vi "Teleop.vi"(10 "Match Info":T1={"Autonomous Elapsed Seconds"=0.0, "TeleOp Elapsed Seconds"=0.0, "Disabled Elapsed Seconds"=0.0, "Visited Autonomous"=FALSE, "Visited TeleOp"=FALSE, "Visited Disabled"=FALSE, "Autonomous Settings"={"Autonomous Style"=enum."Independent", "VI Refnum"=refnum}}, 11 "Call Context":T2) -> ()   [LabVIEW 2017]
doc: "This VI is called for each TeleOp packet received from the DS where the robot is not disabled. It is often used to read from the joysticks and update I/O or to update setpoints for timed control loops. It should complete and return within 20 milliseconds or it may miss DS packets."
uses:
  <vilib>/Rock Robotics/WPI/DriverStation/WPI_DriverStationDerivedRobotMode.ctl
  <vilib>/Rock Robotics/WPI/DriverStation/WPI_DriverStationMatch Info.ctl
  <vilib>/Rock Robotics/WPI/Utilities/WPI_GetSetVariantRefNum.vi
  Globals/Driver Controller Inputs.vi
  Globals/Manipulator Controller Inputs.vi
  Globals/Robot Global Data.vi
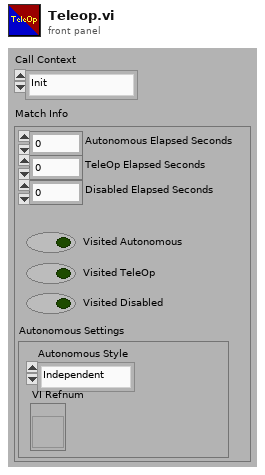
[diagram p1: front panel]
types:
  T1 = typedef "WPI_DriverStationMatch Info.ctl" = cluster{"Autonomous Elapsed Seconds":dbl, "TeleOp Elapsed Seconds":dbl, "Disabled Elapsed Seconds":dbl, "Visited Autonomous":bool, "Visited TeleOp":bool, "Visited Disabled":bool, "Autonomous Settings":cluster{"Autonomous Style":enum16{"Iterative", "Independent"}, "VI Refnum":refnum<vi>}}
  T2 = typedef "WPI_DriverStationDerivedRobotMode.ctl" = enum16{"Init", "Execute", "Stop"}
  T3 = typedef "WPI_JoystickDevRef.ctl" = cluster{"Device":T4}
  T4 = typedef "WPI_JoystickDeviceEnum.ctl" = enum16{"USB 0", "USB 1", "USB 2", "USB 3", "USB 4", "USB 5"}
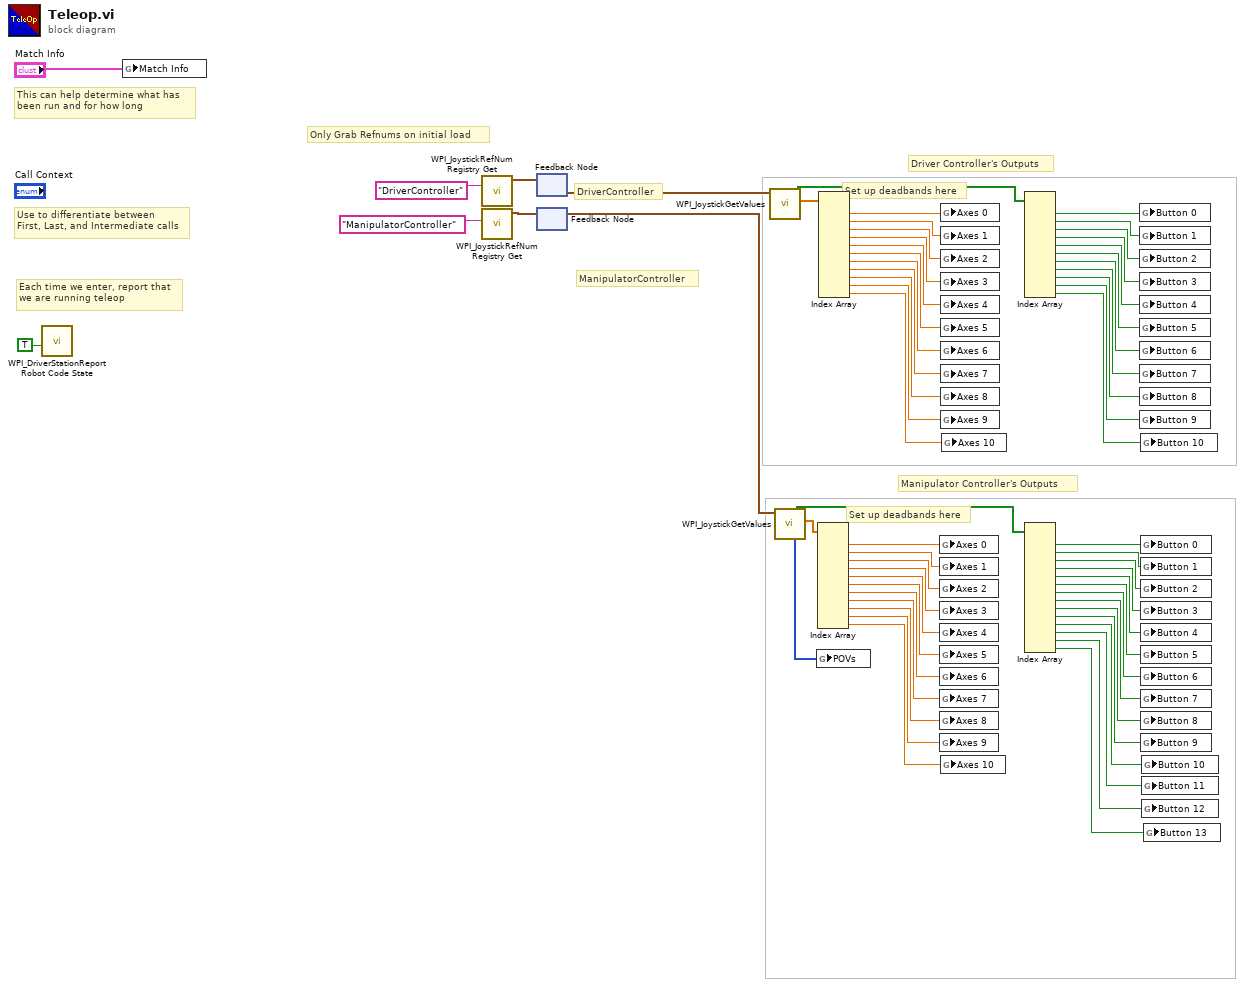
[diagram p0: block diagram]
diagram:
  # "ManipulatorController"
  # "DriverController"
  # "Only Grab Refnums on initial load"
  # "Set up deadbands here"
  # "Set up deadbands here"
  # "Driver Controller's Outputs"
  # "Manipulator Controller's Outputs"
  # "Each time we enter, report that\nwe are running teleop"
  # "Use to differentiate between\nFirst, Last, and Intermediate calls"
  # "This can help determine what has\nbeen run and for how long"
  n1 = call <vilib>:"WPI_DriverStationReport Robot Code State.vi"("TeleOp"=TRUE ("Autonomous")) -> ()  [unwired: 10 in, 1 out]
  n2 = global write "Robot Global Data.vi" "Match Info"("Match Info") -> ()
  n3 = call <vilib>:"WPI_JoystickRefNum Registry Get.vi"("refnum name"="DriverController") -> ("JoystickDevRef"=w9:T3)  [unwired: 1 in, 9 out]
  n4 = call <vilib>:"WPI_JoystickRefNum Registry Get.vi"("refnum name"="ManipulatorController") -> ("JoystickDevRef"=w8:T3)  [unwired: 1 in, 9 out]
  n5 = feedback #1() -> (w35:T3)  [unwired: 1 in]
  n6 = feedback-in #1(w9) -> ()
  n7 = feedback #2() -> (w10:T3)  [unwired: 1 in]
  n8 = feedback-in #2(w8) -> ()
  n9 = call <vilib>:"WPI_JoystickGetValues.vi"("JoystickDevRef"=w35) -> ("Buttons"=w36:bool[], "Axes"=w59:dbl[])  [unwired: 6 in, 3 out]
  n10 = call <vilib>:"WPI_JoystickGetValues.vi"("JoystickDevRef"=w10) -> ("Buttons"=w11:bool[], "Axes"=w34:dbl[], "POVs"=w7:i16[])  [unwired: 6 in, 2 out]
  n11 = global write "Manipulator Controller Inputs.vi" "POVs"(w7) -> ()
  n12 = Index Array(array=w34) -> (element #1=w33:dbl, element #2=w32:dbl, element #3=w31:dbl, element #4=w30:dbl, element #5=w24:dbl, element #6=w23:dbl, element #7=w29:dbl, element #8=w28:dbl, element #9=w27:dbl, element #10=w26:dbl, element #11=w25:dbl)  [unwired: 11 in]
  n13 = Index Array(array=w59) -> (element #1=w58:dbl, element #2=w57:dbl, element #3=w56:dbl, element #4=w55:dbl, element #5=w54:dbl, element #6=w53:dbl, element #7=w52:dbl, element #8=w51:dbl, element #9=w50:dbl, element #10=w49:dbl, element #11=w48:dbl)  [unwired: 11 in]
  n14 = global write "Manipulator Controller Inputs.vi" "Axes 0"(w33) -> ()
  n15 = global write "Manipulator Controller Inputs.vi" "Axes 1"(w32) -> ()
  n16 = global write "Manipulator Controller Inputs.vi" "Axes 2"(w31) -> ()
  n17 = global write "Manipulator Controller Inputs.vi" "Axes 3"(w30) -> ()
  n18 = global write "Manipulator Controller Inputs.vi" "Axes 4"(w24) -> ()
  n19 = global write "Manipulator Controller Inputs.vi" "Axes 5"(w23) -> ()
  n20 = global write "Manipulator Controller Inputs.vi" "Axes 6"(w29) -> ()
  n21 = global write "Manipulator Controller Inputs.vi" "Axes 7"(w28) -> ()
  n22 = global write "Manipulator Controller Inputs.vi" "Axes 8"(w27) -> ()
  n23 = global write "Manipulator Controller Inputs.vi" "Axes 9"(w26) -> ()
  n24 = global write "Driver Controller Inputs.vi" "Axes 0"(w58) -> ()
  n25 = global write "Driver Controller Inputs.vi" "Axes 1"(w57) -> ()
  n26 = global write "Driver Controller Inputs.vi" "Axes 2"(w56) -> ()
  n27 = global write "Driver Controller Inputs.vi" "Axes 3"(w55) -> ()
  n28 = global write "Driver Controller Inputs.vi" "Axes 4"(w54) -> ()
  n29 = global write "Driver Controller Inputs.vi" "Axes 5"(w53) -> ()
  n30 = global write "Driver Controller Inputs.vi" "Axes 6"(w52) -> ()
  n31 = global write "Driver Controller Inputs.vi" "Axes 7"(w51) -> ()
  n32 = global write "Driver Controller Inputs.vi" "Axes 8"(w50) -> ()
  n33 = global write "Driver Controller Inputs.vi" "Axes 9"(w49) -> ()
  n34 = global write "Manipulator Controller Inputs.vi" "Axes 10"(w25) -> ()
  n35 = global write "Driver Controller Inputs.vi" "Axes 10"(w48) -> ()
  n36 = Index Array(array=w36) -> (element #1=w37:bool, element #2=w38:bool, element #3=w39:bool, element #4=w40:bool, element #5=w41:bool, element #6=w42:bool, element #7=w43:bool, element #8=w44:bool, element #9=w45:bool, element #10=w46:bool, element #11=w47:bool)  [unwired: 11 in]
  n37 = Index Array(array=w11) -> (element #1=w22:bool, element #2=w21:bool, element #3=w20:bool, element #4=w19:bool, element #5=w13:bool, element #6=w12:bool, element #7=w18:bool, element #8=w17:bool, element #9=w16:bool, element #10=w15:bool, element #11=w14:bool, element #12=w5:bool, element #13=w4:bool, element #14=w3:bool)  [unwired: 14 in]
  n38 = global write "Driver Controller Inputs.vi" "Button 0"(w37) -> ()
  n39 = global write "Driver Controller Inputs.vi" "Button 1"(w38) -> ()
  n40 = global write "Driver Controller Inputs.vi" "Button 2"(w39) -> ()
  n41 = global write "Driver Controller Inputs.vi" "Button 3"(w40) -> ()
  n42 = global write "Driver Controller Inputs.vi" "Button 4"(w41) -> ()
  n43 = global write "Driver Controller Inputs.vi" "Button 5"(w42) -> ()
  n44 = global write "Driver Controller Inputs.vi" "Button 6"(w43) -> ()
  n45 = global write "Driver Controller Inputs.vi" "Button 7"(w44) -> ()
  n46 = global write "Driver Controller Inputs.vi" "Button 8"(w45) -> ()
  n47 = global write "Driver Controller Inputs.vi" "Button 9"(w46) -> ()
  n48 = global write "Driver Controller Inputs.vi" "Button 10"(w47) -> ()
  n49 = global write "Manipulator Controller Inputs.vi" "Button 0"(w22) -> ()
  n50 = global write "Manipulator Controller Inputs.vi" "Button 1"(w21) -> ()
  n51 = global write "Manipulator Controller Inputs.vi" "Button 2"(w20) -> ()
  n52 = global write "Manipulator Controller Inputs.vi" "Button 3"(w19) -> ()
  n53 = global write "Manipulator Controller Inputs.vi" "Button 4"(w13) -> ()
  n54 = global write "Manipulator Controller Inputs.vi" "Button 5"(w12) -> ()
  n55 = global write "Manipulator Controller Inputs.vi" "Button 6"(w18) -> ()
  n56 = global write "Manipulator Controller Inputs.vi" "Button 7"(w17) -> ()
  n57 = global write "Manipulator Controller Inputs.vi" "Button 8"(w16) -> ()
  n58 = global write "Manipulator Controller Inputs.vi" "Button 9"(w15) -> ()
  n59 = global write "Manipulator Controller Inputs.vi" "Button 10"(w14) -> ()
  n60 = global write "Manipulator Controller Inputs.vi" "Button 11"(w5) -> ()
  n61 = global write "Manipulator Controller Inputs.vi" "Button 12"(w4) -> ()
  n62 = global write "Manipulator Controller Inputs.vi" "Button 13"(w3) -> ()
